vi "get_average_L.vi"(10 "input2 (int)":i32, 11 "input1 (int)":i32) -> (2 "output2 (int)":dbl, 3 "output1 (int)":dbl)   [LabVIEW 2019]
panel:
  out "output2 (dbl)":dbl
  out "output1 (dbl)":dbl
  out "one shot rising":bool
  in  "Calibration on":bool=TRUE
  out "iteraction":i32
  out "output2 temp(dbl)":dbl
  out "output1 temp (dbl)":dbl
  out "output2 temp (int)":i32
  out "output1 temp (int)":i32
  in  "input2 (dbl)":dbl
  in  "input1 (dbl)":dbl
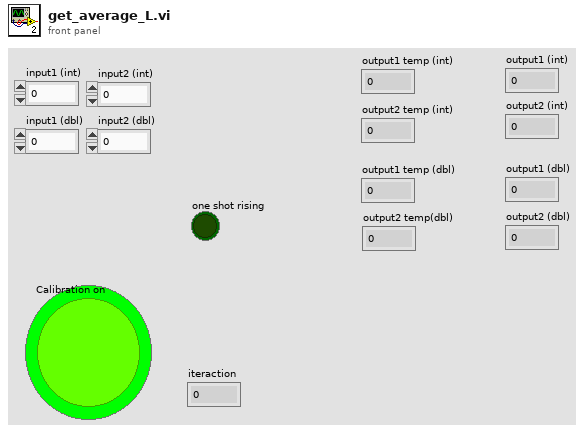
[diagram p1: front panel]
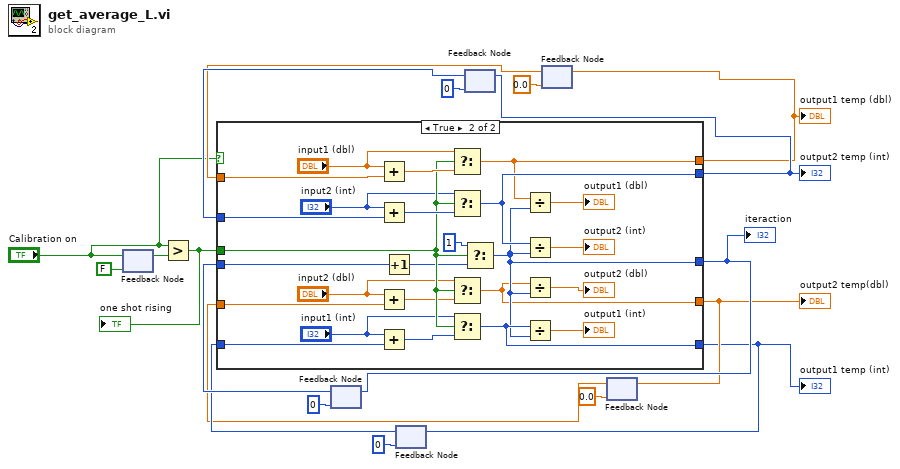
[diagram p0: block diagram]
diagram:
  n1 = feedback #1(FALSE) -> (w4:bool)
  n2 = feedback-in #1("Calibration on") -> ()
  n3 = Greater?(x="Calibration on", y=w4) -> (0:w1:bool)
  "one shot rising" <- w1
  n4 = feedback #2(0) -> (w15:i32)
  n5 = feedback #3(0) -> (w12:i32)
  n6 = feedback #4(0) -> (w11:i32)
  n7 = feedback #5(0.0) -> (w9:dbl)
  n8 = feedback #6(0.0) -> (w7:dbl)
  n9 = case shown="True" "Calibration on" {
    tunnel: w15 -> [w20 w49]
    tunnel: [w20 w26] -> w14
    tunnel: w12 -> [w23 w48]
    tunnel: [w23 w33] -> w5
    tunnel: w11 -> [w24 w47]
    tunnel: [w24 w30] -> w10
    tunnel: w9 -> [w21 w46]
    tunnel: [w21 w28] -> w8
    tunnel: w7 -> [w22 w45]
    tunnel: [w22 w25] -> w6
    tunnel: w1 -> [_ w41]
    frame False {
    }
    frame True {
      n10 = Add(x="input1 (dbl)", y=w46) -> (x+y=w42:dbl)
      n11 = Add(x="input2 (int)", y=w47) -> (x+y=w43:i32)
      n12 = Add(x="input2 (dbl)", y=w45) -> (x+y=w40:dbl)
      n13 = Add(x="input1 (int)", y=w48) -> (x+y=w44:i32)
      n14 = Increment(x=w49) -> (x+1=w39:i32)
      n15 = Select(t="input1 (dbl)", s=w41, f=w42) -> (s? t:f=w28:dbl)
      n16 = Select(t="input2 (int)", s=w41, f=w43) -> (s? t:f=w30:i32)
      n17 = Select(t="input2 (dbl)", s=w41, f=w40) -> (s? t:f=w25:dbl)
      n18 = Select(t="input1 (int)", s=w41, f=w44) -> (s? t:f=w33:i32)
      n19 = Select(t=1, s=w41, f=w39) -> (s? t:f=w26:i32)
      n20 = Divide(x=w28, y=w26) -> (x/y=→"output1 (dbl)":dbl)
      n21 = Divide(x=w30, y=w26) -> (x/y=→"output2 (int)":dbl)
      n22 = Divide(x=w25, y=w26) -> (x/y=→"output2 (dbl)":dbl)
      n23 = Divide(x=w33, y=w26) -> (x/y=→"output1 (int)":dbl)
    }
  }
  "output2 temp (int)" <- w10
  "output1 temp (dbl)" <- w8
  "output2 temp(dbl)" <- w6
  "iteraction" <- w14
  "output1 temp (int)" <- w5
  n24 = feedback-in #2(w14) -> ()
  n25 = feedback-in #3(w5) -> ()
  n26 = feedback-in #4(w10) -> ()
  n27 = feedback-in #5(w8) -> ()
  n28 = feedback-in #6(w6) -> ()
